vi "send PVUpdate.vi"(8 "error in (no error)":errorcluster, 9 "PV":refnum<class "PV.lvclass">, 10 "CS++PVUpdate Msg in":refnum<class "CS++PVUpdate Msg.lvclass">, 11 "Message Enqueuer in":refnum<class "Message Enqueuer.lvclass">) -> (0 "error out":errorcluster, 3 "Message Enqueuer out":refnum<class "Message Enqueuer.lvclass">)   [LabVIEW 2014, in "CS++PVMonitor.lvlib" / "CS++PVUpdate Msg.lvclass"]
uses:
  CS++PVUpdate Msg.lvclass
  Classes/CS++ProcessVariables/ProcessVariable/PV.lvclass
  <vilib>/ActorFramework/Message Enqueuer/Message Enqueuer.lvclass
  CS++PVUpdate Msg.lvclass/CS++PVUpdate Msg.ctl
  Classes/CS++ProcessVariables/ProcessVariable/PV.lvclass/PV.ctl
  <vilib>/ActorFramework/Message Enqueuer/Message Enqueuer.lvclass/Message Enqueuer.ctl
  <vilib>/ActorFramework/Message Priority Queue/Priority Enqueue.vi
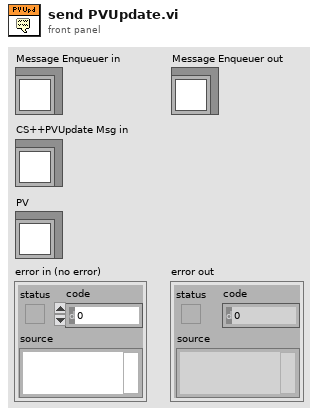
[diagram p1: front panel]
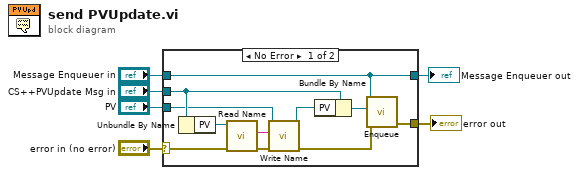
[diagram p0: block diagram]
diagram:
  n1 = case shown="No Error" "error in (no error)" {
    selector: "error in (no error)" -> [w8 w19]
    tunnel: [w16 w19] -> w5
    tunnel: "CS++PVUpdate Msg in" -> [w14 _]
    tunnel: "PV" -> [w12 _]
    tunnel: "Message Enqueuer in" -> [w15 w18]
    tunnel: [w15 w18] -> w1
    frame No Error {
      n2 = Unbundle By Name(w14) -> ("PV"=w13:refnum<class "PV.lvclass">)
      n3 = call "Read Name.vi"("error in (no error)"=w8, "PV in"=w13) -> ("error out"=w10:errorcluster, "Name"=w9:string)  [unwired: 7 in, 1 out]
      n4 = call "Write Name.vi"("error in (no error)"=w10, "Name"=w9, "PV in"=w12) -> ("error out"=w7:errorcluster, "PV out"=w11:refnum<class "PV.lvclass">)  [unwired: 7 in]
      n5 = Bundle By Name(cluster=w14, "PV"=w11) -> (w17:refnum<class "CS++PVUpdate Msg.lvclass">)
      n6 = call <vilib>:"Enqueue.vi"("error in (no error)"=w7, "Message"=w17, "Message Enqueuer in"=w15) -> ("error out"=w16:errorcluster)  [unwired: 7 in, 1 out]
    }
    frame Error {
    }
  }
  "error out" <- w5
  "Message Enqueuer out" <- w1
